vi "Create.vi"(5 "Is Same Type in":refnum<class "Is Same Type.lvclass">, 8 "error in (no error)":errorcluster, 11 "Expected":variant) -> (0 "error out":errorcluster, 3 "Is Same Type":refnum<class "Is Same Type.lvclass">)   [LabVIEW 2017, in "Transparent Assertions.lvlib" / "Is Same Type.lvclass"]
uses:
  Is Same Type.lvclass
  Is Same Type.lvclass/Is Same Type.ctl
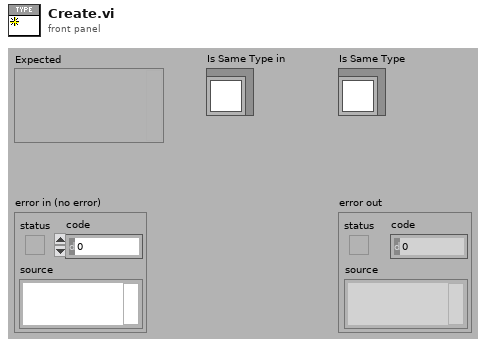
[diagram p1: front panel]
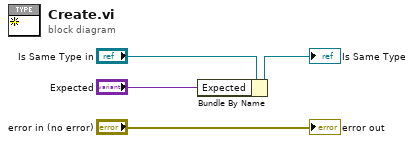
[diagram p0: block diagram]
diagram:
  n1 = Bundle By Name(cluster="Is Same Type in", "Expected"="Expected") -> (→"Is Same Type":refnum<class "Is Same Type.lvclass">)
  "error out" <- "error in (no error)"
